vi "PAS IO.vi"   [LabVIEW 2015]
uses:
  <vilib>/Platform/TimedLoop/XDataNode/timing_clust.ctl
  <vilib>/Platform/TimedLoop/XDataNode/nitl_modes.ctl
  <vilib>/Platform/TimedLoop/XDataNode/wakeup.ctl
  <vilib>/rvi/Emulation/niFpgaGetClockAttributes.vi
  <vilib>/rvi/Emulation/niFpgaSctlEmulationGetInTimedLoop.vi
  <vilib>/rvi/Emulation/niFpgaEmulationReportErrorSimple.vi
  <vilib>/rvi/Emulation/niFpgaEmulationIsFPGAContextNoSignature.vi
  <vilib>/rvi/DataTransferAndStorage/Container/Common/niFpgaContainerGetUniqueNameForEmu.vi
  <vilib>/rvi/Memory/Memory_Emulation/niFpgaMemoryEmulationCacheClearOnFirstRun.vi
  <vilib>/rvi/Memory/Memory_Emulation/nirvimemoryEmulationManagerCache_MakeExclusive.vi
  <vilib>/rvi/Memory/Memory_Emulation/niFpgaMemoryEmulationValidateCache.vi
  <vilib>/rvi/Memory/Memory_Emulation/nirvimemoryEmulationManagerCache_InsertValue.vi
  <vilib>/Utility/error.llb/Clear Errors.vi
  <vilib>/rvi/Memory/Memory_Emulation/nirvimemoryEmulationManagerCache_ReleaseExclusive.vi
  <vilib>/rvi/Memory/Memory_Emulation/nirvimemoryEmulationManagerCache_GetValue.vi
  <vilib>/rvi/Memory/Memory_Emulation/nirvimemoryEmulationManagerCache_SetValue.vi
  <vilib>/rvi/Emulation/niFpgaProcessEmulError.vi
  <vilib>/rvi/eio/common/nirviEmuTemplateMethod_errors.vi
  <vilib>/rvi/interface/RandomDataEmulation/niFpgaRandomDataHandleErrors.vi
  <vilib>/rvi/Emulation/niFpgaCriticalErrorInLSC.vi
  <vilib>/rvi/Memory/Memory_Emulation/nirvimemoryFastEmulation.vi
  <vilib>/rvi/Memory/Memory_Emulation/nirvimemoryEmulation.vi
  <vilib>/rvi/errors/nirviReportUnexpectedCaseInternalError (U32).vi
  <vilib>/rvi/DataTransferAndStorage/Container/XNode/niFpgaContainer.xnode
  <vilib>/rvi/DataTransferAndStorage/Register/Emulation/niFpgaRegisterEmulation.vi
  <vilib>/eio/EIONode/EIONode.xnode
  <vilib>/rvi/interface/RandomDataEmulation/nirviRandomDataFpgaReadWriteTemplate.vi
  <vilib>/rvi/FXPMathLib/FxpMul/XNode/nifxpmath_Multiplier.xnode
  <vilib>/rvi/FXPMathLib/FxpAdd/XNode/nifxpmath_Add.xnode
  <vilib>/Platform/TimedLoop/XDataNode/XDataNode.xnode
  <vilib>/rvi/FXPMathLib/sim/FxpSim.dll
  <vilib>/Platform/TimedLoop/XDataNode/XDNodeRunTimeDep.lvlib
types:
  T1 = typedef "XDNodeRunTimeDep.lvlib/timing_clust.ctl" = cluster{"Expected End [f-1]":u64, "Actual End [f-1]":u64, "Finished Late? [f-1]":bool, "Expected End [i-1]":u64, "Actual End [i-1]":u64, "Finished Late? [i-1]":bool, "Expected Start [i]":u64, "Actual Start [i]":u64, "Expected Start [f]":u64, "Actual Start [f]":u64, "Source Name":string, "Structure Name":string, "Period":i64, "Deadline":i64, "Offset":i64, "Start":i64, "Priority":i32, "Timeout":i32, "Mode":T2, "Wakeup Reason":T3, "Error":errorcluster, "Source Type":string, "Secondary Source Type":string, "Global End Time":u64, "Global Start Time":u64, "Frame Duration":u64, "Iteration Duration":u64, "Assigned CPU":i32, "I/O Scan Engine Mode":u32}
  T2 = typedef "XDNodeRunTimeDep.lvlib/nitl_modes.ctl" = enum32{"No Change", "Process missed periods, maintain original phase", "Discard missed periods, maintain original phase", "Process missed periods, ignore original phase", "Discard missed periods, ignore original phase"}
  T3 = typedef "XDNodeRunTimeDep.lvlib/wakeup.ctl" = enum32{"Normal", "Aborted", "Asynchronous wakeup", "Timing source error", "Timed loop error", "Timeout"}
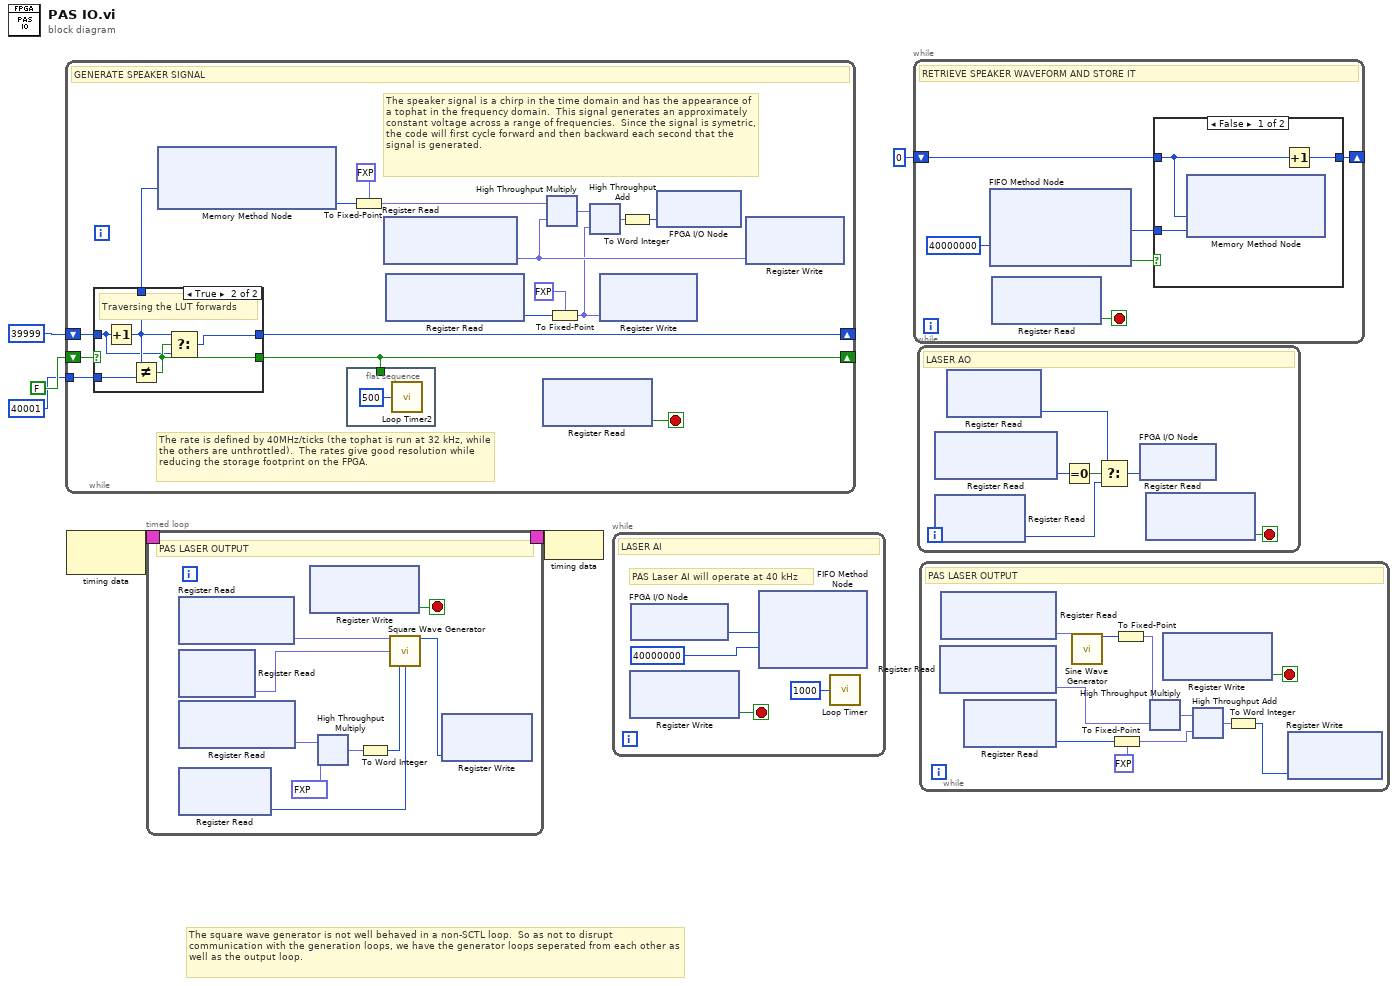
[diagram p0: block diagram]
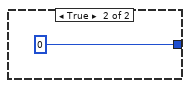
[diagram p2: hidden frame]
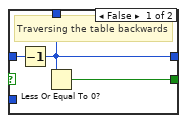
[diagram p3: hidden frame]
diagram:
  # "The square wave generator is not well behaved in a non-SCTL loop.  So as not to disrupt communication with the generation loops, we have the generator loops seperated from each other as well as the output loop."
  n1 = while {
    shift-right: [w18] -> _
    shift-left: FALSE -> [w23]
    shift-right: [w19] -> _
    shift-left: u32 39999 -> [w20]
    tunnel: u32 40001 ("y") -> [w21]
    stop <- w17 stop-if-true
    # "The rate is defined by 40MHz/ticks (the tophat is run at 32 kHz, while the others are unthrottled).  The rates give good resolution while reducing the storage footprint on the FPGA."
    # "The speaker signal is a chirp in the time domain and has the appearance of a tophat in the frequency domain.  This signal generates an approximately constant voltage across a range of frequencies.  Since the signal is symetric, the code will first cycle forward and then backward each second that the signal is generated."
    # "GENERATE SPEAKER SIGNAL"
    n2 = case "Check where we are in the chirp" shown="True" w23 {
      tunnel: w20 -> [w27 w28]
      tunnel: [w26 w31] -> w18
      tunnel: [w25 w32] -> w14
      tunnel: w21 -> [_ w30]
      tunnel: [w25 w29] -> w19
      frame False {
        # "Traversing the table backwards"
        n3 = Decrement(x=w27) -> (x-1=w25:u32)
        n4 = Less Or Equal To 0?(x=w25) -> (x <= 0?=w26:bool)
      }
      frame True {
        # "Traversing the LUT forwards"
        n5 = Increment(x=w28) -> (x+1=w32:u32)
        n6 = Not Equal?(x=w32, y=w30) -> (x != y?=w31:bool)
        n7 = Select(t=w32, s=w31, f=w28) -> (s? t:f=w29:u32)
      }
    }
    n8 = xnode ("Memory Method Node")("Address"=w14) -> ("Data"=w13:i16)  [unwired: 1 in, 1 out]
    n9 = flat-sequence {
      tunnel: w18 -> [_]
      frame #0 {
        n10 = call "Loop Timer2"("Count(Ticks)"=u32 500) -> ()  [unwired: 1 out]
      }
    }
    n11 = To Fixed-Point(fixed-point type=fxp<+/-,16,16> 0.0, number=w13) -> (fixed-point=w12:fxp<+/-,16,16>)
    n12 = xnode ("Register Read")() -> ("Data"=w9:fxp<+,32,0>)  [unwired: 1 in, 1 out]
    n13 = xnode ("Register Read")() -> ("Data"=w8:i16)  [unwired: 1 in, 1 out]
    n14 = xnode ("Register Read")() -> ("Data"=w17:bool)  [unwired: 1 in, 1 out]
    n15 = xnode ("High Throughput Multiply")("x"=w12, "y"=w9) -> ("x*y"=w22:fxp<+/-,16,16>)
    n16 = To Fixed-Point(fixed-point type=fxp<+/-,16,16> 0.0, number=w8) -> (fixed-point=w7:fxp<+/-,16,16>)
    n17 = xnode ("High Throughput Add")("x"=w22, "y"=w7) -> ("x+y"=w16:fxp<+/-,16,16>)
    n18 = xnode ("Register Write")("Data"=w7) -> ()  [unwired: 1 in, 1 out]
    n19 = To Word Integer(number=w16) -> (16bit integer=w15:i16)
    n20 = xnode "FPGA I/O Node"("Speaker"=w15) -> ()  [unwired: 1 in, 1 out]
    n21 = xnode ("Register Write")("Data"=w9) -> ()  [unwired: 1 in, 1 out]
  }
  n22 = node-c288() -> (w3:T1)  [unwired: 1 in]
  n23 = timed-loop "Square wave generation - SCTL" {
    timing: w3 -> [_]
    timing-out: [_] -> w2
    stop <- w41 stop-if-true
    # "PAS LASER OUTPUT"
    n24 = xnode ("Register Read")() -> ("Data"=w40:fxp<+,32,0>)  [unwired: 1 in, 1 out]
    n25 = xnode ("Register Read")() -> ("Data"=w34:fxp<+,32,0>)  [unwired: 1 in, 1 out]
    n26 = xnode ("Register Read")() -> ("Data"=w38:fxp<+,32,0>)  [unwired: 1 in, 1 out]
    n27 = xnode ("Register Read")() -> ("Data"=w39:i16)  [unwired: 1 in, 1 out]
    n28 = xnode ("Register Write")() -> ("Data"=w41:bool)  [unwired: 1 in, 1 out]
    n29 = xnode ("High Throughput Multiply")("x"=w38, "y"=fxp<+,16,16> 32767.0) -> ("x*y"=w36:fxp<+/-,16,16>)
    n30 = To Word Integer(number=w36) -> (16bit integer=w35:i16)
    n31 = call "Square Wave Generator"("frequency (periods/tick)"=w40, "duty cycle (periods)"=w34, "amplitude"=w35, "offset"=w39) -> ("square wave out"=w33:i16)  [unwired: 11 in]
    n32 = xnode "Register Write"("Data"=w33) -> ()  [unwired: 1 in, 1 out]
  }
  n33 = node-c288(w2) -> ()
  n34 = while {
    stop <- w47 stop-if-true
    # "PAS Laser AI will operate at 40 kHz"
    # "LASER AI"
    n35 = xnode ("Register Write")() -> ("Data"=w47:bool)  [unwired: 1 in, 1 out]
    n36 = xnode "FPGA I/O Node"() -> ("PAS Las In"=w46:i16)  [unwired: 1 in, 1 out]
    n37 = xnode ("FIFO Method Node")("Element"=w46, "Timeout"=40000000) -> ()  [unwired: 1 in, 2 out]
    n38 = call "Loop Timer"("Count(Ticks)"=u32 1000) -> ()  [unwired: 1 out]
  }
  n39 = while {
    shift-right: [w48] -> _
    shift-left: u32 0 ("Address") -> [w49]
    stop <- w50 stop-if-true
    # "RETRIEVE SPEAKER WAVEFORM AND STORE IT"
    n40 = xnode ("FIFO Method Node")("Timeout"=40000000) -> ("Element"=w51:i16, "Timed Out?"=w52:bool)  [unwired: 1 in, 1 out]
    n41 = xnode ("Register Read")() -> ("Data"=w50:bool)  [unwired: 1 in, 1 out]
    n42 = case shown="False" w52 {
      tunnel: w51 -> [w56 _]
      tunnel: w49 -> [w54 _]
      tunnel: [w55 u32 0 ("Address")] -> w48
      frame False {
        n43 = xnode ("Memory Method Node")("Address"=w54, "Data"=w56) -> ()  [unwired: 1 in, 1 out]
        n44 = Increment(x=w54) -> (x+1=w55:u32)
      }
      frame True {
      }
    }
  }
  n45 = while {
    stop <- w63 stop-if-true
    # "LASER AO"
    n46 = xnode ("Register Read")() -> ("Data"=w62:u8)  [unwired: 1 in, 1 out]
    n47 = xnode "Register Read"() -> ("Data"=w59:i16)  [unwired: 1 in, 1 out]
    n48 = xnode "Register Read"() -> ("Data"=w58:i16)  [unwired: 1 in, 1 out]
    n49 = Equal To 0?(x=w62) -> (x = 0?=w61:bool)
    n50 = Select(t=w58, s=w61, f=w59) -> (s? t:f=w60:i16)
    n51 = xnode "FPGA I/O Node"("Laser"=w60) -> ()  [unwired: 1 in, 1 out]
    n52 = xnode ("Register Read")() -> ("Data"=w63:bool)  [unwired: 1 in, 1 out]
  }
  n53 = while "Square wave generation - SCTL" {
    stop <- w74 stop-if-true
    # "PAS LASER OUTPUT"
    n54 = xnode ("Register Read")() -> ("Data"=w67:fxp<+,32,0>)  [unwired: 1 in, 1 out]
    n55 = xnode ("Register Read")() -> ("Data"=w68:fxp<+,32,0>)  [unwired: 1 in, 1 out]
    n56 = xnode ("Register Read")() -> ("Data"=w66:i16)  [unwired: 1 in, 1 out]
    n57 = call "Sine Wave Generator"("frequency (periods/tick)"=w68) -> ("sine out"=w73:i16)  [unwired: 14 in]
    n58 = To Fixed-Point(fixed-point type=fxp<+/-,16,16> 0.0, number=w66) -> (fixed-point=w70:fxp<+/-,16,16>)
    n59 = To Fixed-Point(number=w73) -> (fixed-point=w72:fxp<+/-,16,16>)  [unwired: 1 in]
    n60 = xnode ("High Throughput Multiply")("x"=w72, "y"=w67) -> ("x*y"=w71:fxp<+/-,16,16>)
    n61 = xnode ("Register Write")() -> ("Data"=w74:bool)  [unwired: 1 in, 1 out]
    n62 = xnode ("High Throughput Add")("x"=w71, "y"=w70) -> ("x+y"=w69:fxp<+/-,16,16>)
    n63 = To Word Integer(number=w69) -> (16bit integer=w64:i16)
    n64 = xnode "Register Write"("Data"=w64) -> ()  [unwired: 1 in, 1 out]
  }
